vi "testNestedEmptyElement.vi"(8 "error in (no error)":errorcluster, 11 "reference in":refnum<class "EasyXML_XML_Subset_Source_Tests.lvclass">) -> (0 "error out":errorcluster, 3 "reference in":refnum<class "EasyXML_XML_Subset_Source_Tests.lvclass">)   [LabVIEW 2013, in "EasyXML_XML_Subset_Source_Tests.lvclass"]
uses:
  EasyXML_XML_Subset_Source_Tests.lvclass
  EasyXML_XML_Subset_Evaluations/EasyXML_XML_Subset_Evaluations.lvclass
panel:
  in  "a":cluster{"b":cluster{"a":string}}
  out "a":cluster{"b":cluster{"a":string}}
  in  "XML String":string="<a>\n  <b>\n    <a/>\n  </b>\n</a>"
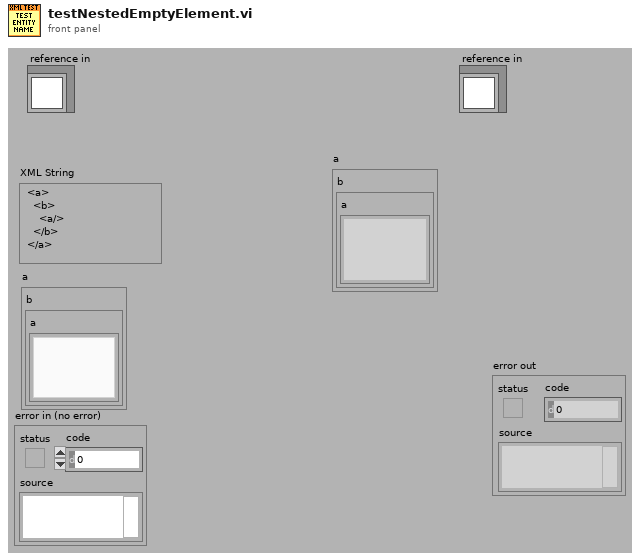
[diagram p1: front panel]
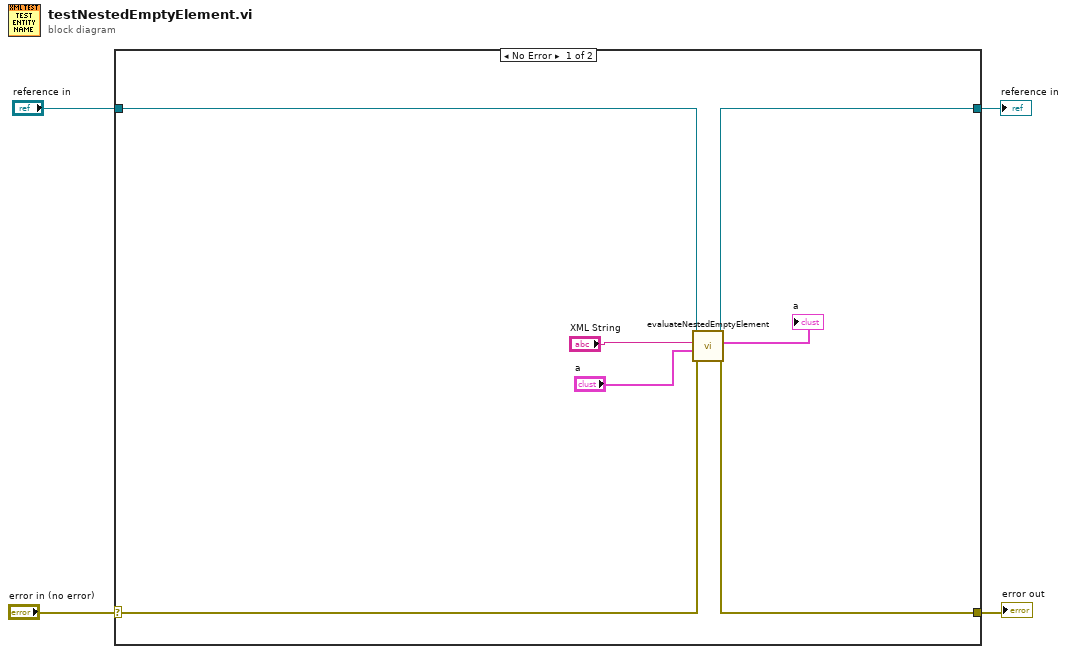
[diagram p0: block diagram]
diagram:
  n1 = case shown="No Error" "error in (no error)" {
    selector: "error in (no error)" -> [w10 w13]
    tunnel: [w8 w13] -> w3
    tunnel: [w11 w12] -> w1
    tunnel: "reference in" -> [w6 w12]
    frame No Error {
      n2 = call "evaluateNestedEmptyElement.vi"("error in (no error)"=w10, "a"="a", "XML String"="XML String", "reference in"=w6) -> ("error out"=w8:errorcluster, "a"=→"a":cluster{"b":cluster{"a":string}}, "reference in"=w11:refnum<class "EasyXML_XML_Subset_Source_Tests.lvclass">)  [unwired: 5 in]
    }
    frame Error {
    }
  }
  "error out" <- w3
  "reference in" <- w1
